vi "Wrap Actor.vi"() -> ()   [LabVIEW 2020, in "Wrapped Actor.lvlib"]
uses:
  Wrapped Actor.lvlib
  Generator/Generator.lvclass
  C:/Program Files/National Instruments/LabVIEW 2020/vi.lib/ActorFramework/Actor/Actor.lvclass
  Source/Actor Pub Sub Channels/Pub Sub Event Channel/Pub Sub Event Channel.lvclass
  E:/Labview/LV 2020/Libs/Actor Pub Sub/Source/Actor Pub Sub Channels/Pub Sub Message Channel/Pub Sub Message Channel.lvclass
  Generator/Generator.lvclass/Generator.ctl
  Source/Actor Pub Sub Channels/Pub Sub Event Channel/Pub Sub Event Channel.lvclass/Pub Sub Event Channel.ctl
  <vilib>/ActorFramework/Message Enqueuer/Message Enqueuer.lvclass/Message Enqueuer.ctl
  Data Message/Data Message.lvclass
  Data Message/Data Message.lvclass/Data Message.ctl
  Data Message/Read Value.vi
  Source/Actor Pub Sub Channels/Pub Sub Event Channel/Read New Message Event.vi
  Generator/Write Result Receiver.vi
  <vilib>/ActorFramework/Message Enqueuer/Enqueue.vi
  <vilib>/ActorFramework/Stop Msg/Stop Msg.lvclass
  C:/Program Files/National Instruments/LabVIEW 2020/vi.lib/ActorFramework/Message/Message.lvclass
  <vilib>/ActorFramework/Message Priority Queue/Priority Enqueue.vi
  <vilib>/ActorFramework/Message/Message.lvclass
  <vilib>/ActorFramework/Actor/Actor.lvclass
  Source/Actor Pub Sub Channels/Pub Sub Message Channel/Pub Sub Message Channel.lvclass
panel:
  in  "stop":bool
  out "Waveform Chart":dbl(graph)
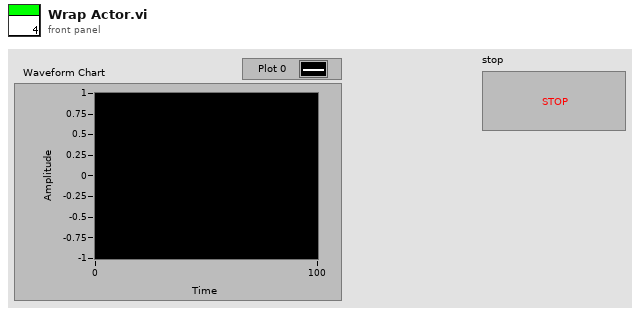
[diagram p1: front panel]
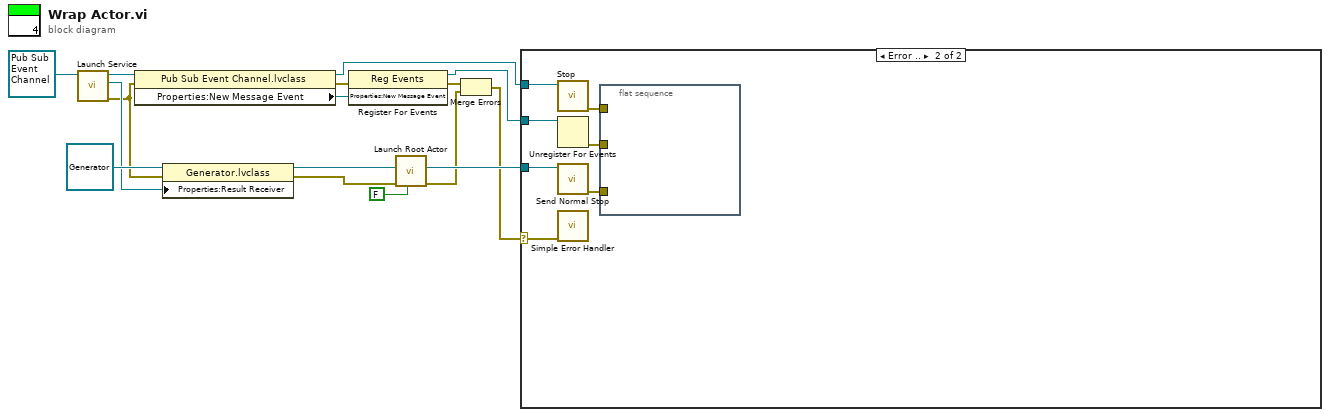
[diagram p0: block diagram]
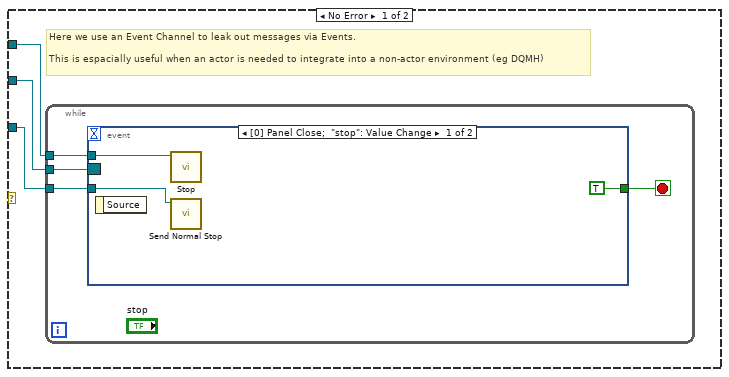
[diagram p2: hidden frame]
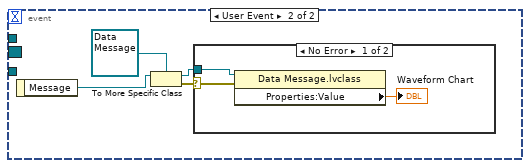
[diagram p3: hidden frame]
diagram:
  n1 = call "Launch Service.vi"("Pub Sub Message Channel"=refnum<class "Pub Sub Event Channel.lvclass"> refnum ("Actor Pub Sub Channels.lvlib:Pub Sub Event Channel.lvclass")) -> ("error out"=w4:errorcluster, "Enqueuer"=w5:refnum<class "Message Enqueuer.lvclass">, "Pub Sub Message Channel Out"=w8:refnum<class "Pub Sub Event Channel.lvclass">)  [unwired: 8 in]
  n2 = property class="Pub Sub Event Channel.lvclass"(reference=w8, error in=w4) -> (reference out=w6:refnum<class "Pub Sub Event Channel.lvclass">, error out=w7:errorcluster, "Properties:New Message Event"=w14:refnum<user-event>)
  n3 = property class="Generator.lvclass"(reference=refnum<class "Generator.lvclass"> refnum ("Wrapped Actor.lvlib:Generator.lvclass"), error in=w4, "Properties:Result Receiver"=w5) -> (reference out=w15:refnum<class "Generator.lvclass">, error out=w12:errorcluster)
  n4 = register-events(error in=w7, w14) -> (reference out=w13:refnum<event-registration>, error out=w3:errorcluster)  [unwired: 1 in]
  n5 = call <vilib>:"Launch Root Actor.vi"("Open Actor Core front panel? (F)"=FALSE, "error in (no error)"=w12, "Actor"=w15) -> ("error out"=w2:errorcluster, "Actor's Enqueuer"=w11:refnum<class "Message Enqueuer.lvclass">)  [unwired: 7 in]
  n6 = Merge Errors(w3, w2) -> (w1:errorcluster)
  n7 = case shown="Error .." w1 {
    selector: w1 -> [_ w34]
    tunnel: w13 -> [w19 w38]
    tunnel: w11 -> [w18 w40]
    tunnel: w6 -> [w17 w39]
    frame No Error {
      # "Here we use an Event Channel to leak out messages via Events.\n\nThis is espacially useful when an actor is needed to integrate into a non-actor environment (eg DQMH)"
      n8 = while {
        tunnel: w19 -> [w23]
        tunnel: w18 -> [w22]
        tunnel: w17 -> [w20]
        stop <- w21 stop-if-true
        n9 = event shown="[0] Panel Close;  \"stop\": Value Change" {
          selector: w23 -> [_ _]
          dyn-events: _ -> [_ _]
          timeout: _ -> [_ _]
          tunnel: w22 -> [w26 _]
          tunnel: [TRUE _] -> w21
          tunnel: w20 -> [w24 _]
          event Panel Close; "stop": Value Change {
            n10 = event-data() -> ()  [unwired: 1 in, 1 out]
            n11 = call "Stop.vi"("Pub Sub Message Channel in"=w24) -> ()  [unwired: 9 in, 2 out]
            n12 = call <vilib>:"Send Normal Stop.vi"("Message Enqueuer"=w26) -> ()  [unwired: 10 in, 1 out]
          }
          event User Event {
            n13 = event-data() -> ("Message"=w30:refnum<class "Message.lvclass">)  [unwired: 1 in]
            n14 = To More Specific Class(target class=refnum<class "Data Message.lvclass"> refnum ("Wrapped Actor.lvlib:Data Message.lvclass"), reference=w30) -> (specific class reference=w27:refnum<class "Data Message.lvclass">, error out=w28:errorcluster)  [unwired: 1 in]
            n15 = case shown="No Error" w28 {
              selector: w28 -> [w33 _]
              tunnel: w27 -> [w32 _]
              frame No Error {
                n16 = property class="Data Message.lvclass"(reference=w32, error in=w33) -> ("Properties:Value"=→"Waveform Chart":dbl)  [unwired: 2 out]
              }
              frame Error {
              }
            }
          }
        }
      }
    }
    frame Error {
      n17 = call "Stop.vi"("Pub Sub Message Channel in"=w39) -> ("error out"=w37:errorcluster)  [unwired: 9 in, 1 out]
      n18 = Unregister For Events(event registration refnum=w38) -> (error out=w36:errorcluster)  [unwired: 1 in]
      n19 = call <vilib>:"Send Normal Stop.vi"("Message Enqueuer"=w40) -> ("error out"=w35:errorcluster)  [unwired: 10 in]
      n20 = call <vilib>:"Simple Error Handler.vi"("error in (no error)"=w34) -> ()  [unwired: 4 in, 5 out]
      n21 = flat-sequence {
        tunnel: w37 -> [_]
        tunnel: w36 -> [_]
        tunnel: w35 -> [_]
        frame #0 {
        }
      }
    }
  }
